vi "fit1.vi"(0 "array":dbl[][](array[numeric]), 5 "num X samples":i32=100, 7 "num Y samples":i32=50, 9 "parameter bounds":T1={"parameter minimum"=[1.0, 0.0, 1.0, 0.0, 1.0, 0.0], "parameter maximum"=[255.0, 640.0, 40.0, 480.0, 40.0, 128.0]}) -> (2 "number of function calls":i32, 3 "Time":u32, 4 "best nonlinear fit":dbl[](array[numeric]), 6 "best fit parameters":dbl[](array[numeric]), 10 "residue":dbl, 14 "estimated parameters":dbl[](array[numeric]), 15 "error out":errorcluster)   [LabVIEW 2015]
uses:
  <vilib>/Analysis/6fits.llb/Curve Fitting Criteria.ctl
  <vilib>/Analysis/1siggen.llb/Ramp Pattern by Samples.vi
  <vilib>/gmath/NumericalOptimization/Nonlinear Curve Fit LM bound.vi
  <vilib>/Analysis/NI_AALBase.lvlib
  <vilib>/gmath/NI_Gmath.lvlib
  <vilib>/Analysis/NI_AALPro.lvlib
panel:
  in  "initial Sigma":dbl=5.0
  out "1D data and fit":dbl[][](graph)
  out "fit param size":i32
  out "Y size":i32
  out "size(bild)":i32[](array[numeric])
  in  "error in (no error)":errorcluster
  in  "termination":cluster{"max iteration":i32, "tolerance":dbl}={"max iteration"=200, "tolerance"=1e-08}
  # "Amplitude"
  # "m1 (Mean 1)"
  # "Sigma 1"
  # "m2 (Mean 2)"
  # "Sigma 2"
  # "Offset"
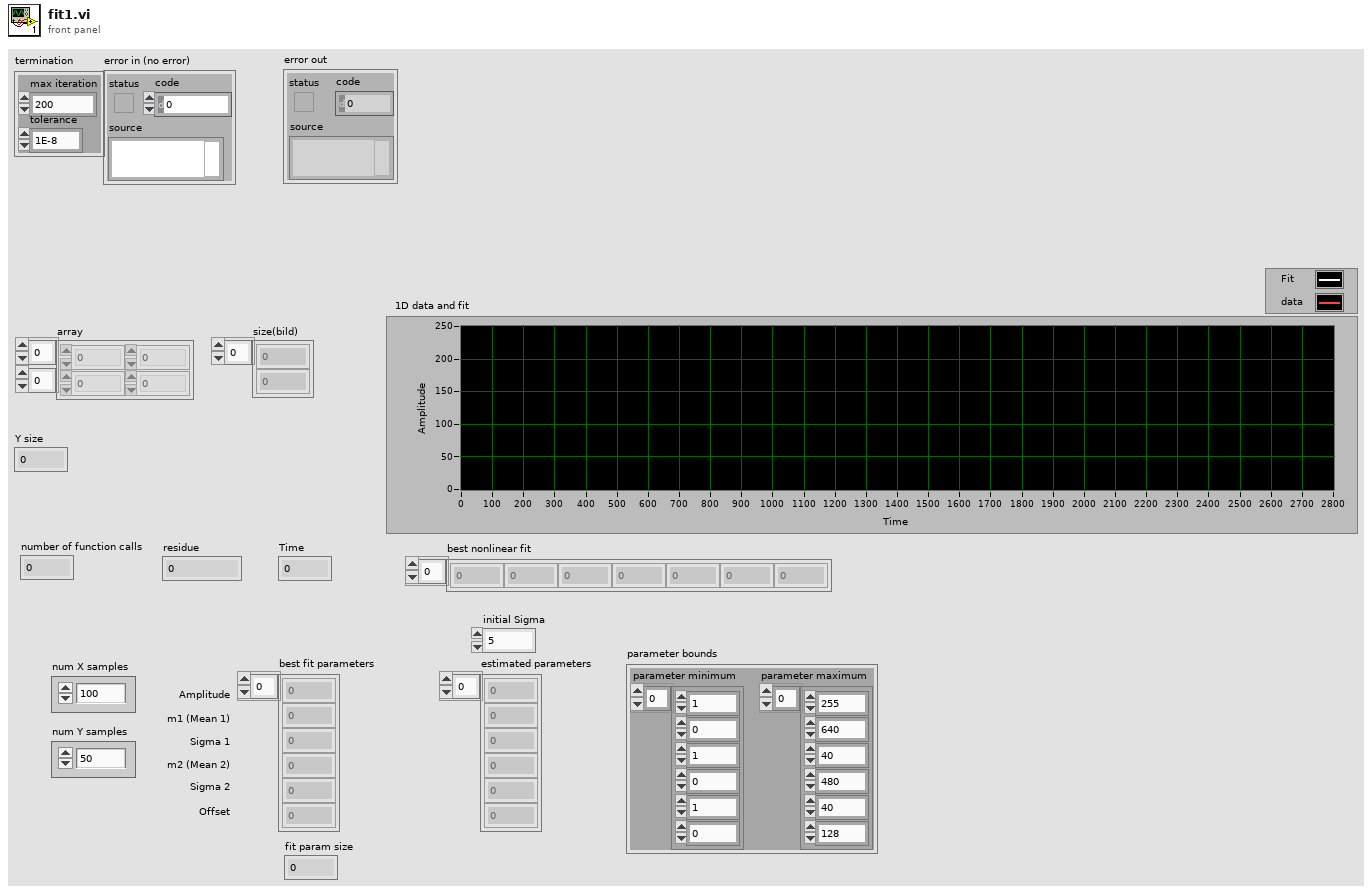
[diagram p1: front panel]
types:
  T1 = cluster{"parameter minimum":dbl[], "parameter maximum":dbl[]}
  T2 = typedef "NI_AALPro.lvlib/Curve Fitting Criteria.ctl" = u16
  T3 = cluster{"num X samples":i32, "num Y samples":i32}
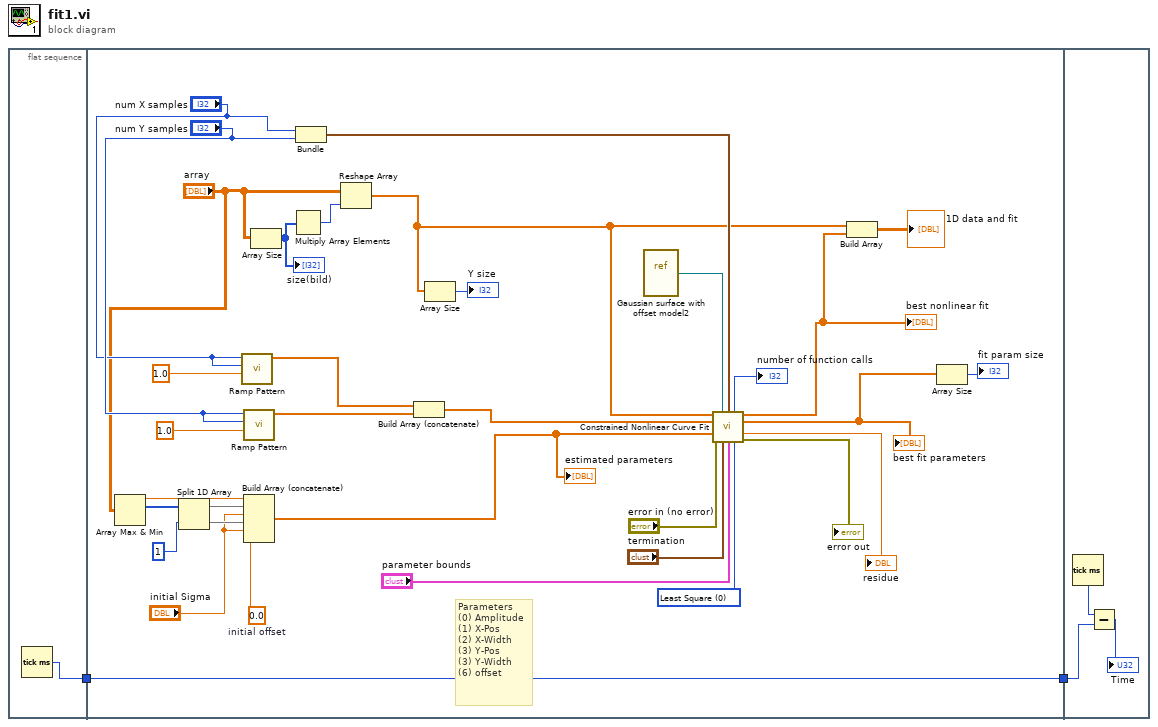
[diagram p0: block diagram]
diagram:
  n1 = flat-sequence {
    tunnel: [w3] -> w2
    tunnel: w2 -> [w37]
    tunnel: [w37] -> w1
    tunnel: w1 -> [w39]
    frame #0 {
      n2 = Tick Count (ms)() -> (millisecond timer value=w3:u32)
    }
    frame #1 {
      w6 = 0.0  # initial offset
      w19 = T2 0 items=["Least Square", "Least Absolute Residual", "Bisquare"] ("method")
      # "Parameters\n(0) Amplitude\n(1) X-Pos\n(2) X-Width\n(3) Y-Pos\n(3) Y-Width\n(6) offset"
      n3 = Array Max & Min(array="array") -> (max value=w13:dbl, max index (indices)=w10:i32[])  [unwired: 2 out]
      n4 = Split 1D Array(array=w10, index=1) -> (first subarray=w9:i32[], second subarray=w8:i32[])
      n5 = call-poly <vilib>:"Ramp Pattern.vi"("start"=1.0, "end"="num X samples", "samples"="num X samples") -> ("Ramp Pattern"=w36:dbl[])  [unwired: 7 in, 1 out]
      n6 = call-poly <vilib>:"Ramp Pattern.vi"("start"=1.0, "end"="num Y samples", "samples"="num Y samples") -> ("Ramp Pattern"=w35:dbl[])  [unwired: 7 in, 1 out]
      n7 = Build Array (concatenate)(w13, w9, "initial Sigma", w8, "initial Sigma", w6) -> (w5:dbl[])
      "estimated parameters" <- w5
      n8 = Array Size(array="array") -> (size(s)=w18:i32[])
      "size(bild)" <- w18
      n9 = Multiply Array Elements(1:w18) -> (0:w17:i32)
      n10 = Bundle("num X samples"="num X samples", "num Y samples"="num Y samples") -> (w24:T3)  [unwired: 1 out]
      n11 = Reshape Array("array", w17) -> (w15:dbl[])
      n12 = Build Array (concatenate)(w36, w35) -> (w20:dbl[])
      n13 = Array Size(array=w15) -> (size(s)=→"Y size":i32)
      n14 = vi-ref "Gaussian surface with offset model2.vi"() -> (w21:refnum<vi>)
      n15 = call-poly <vilib>:"Constrained Nonlinear Curve Fit.vi"("Y"=w15, "f(x,a)"=w21, "data"=w24, "X"=w20, "initial parameters"=w5, "error in (no error)"="error in (no error)", "termination"="termination", "parameter bounds"="parameter bounds", "method"=w19) -> ("number of function calls"=→"number of function calls":i32, "best nonlinear fit"=w14:dbl[], "best fit parameters"=w29:dbl[], "residue"=→"residue":dbl, "error out"=→"error out":errorcluster)  [unwired: 1 in, 1 out]
      "best fit parameters" <- w29
      "best nonlinear fit" <- w14
      n16 = Build Array(w15, w14) -> (→"1D data and fit":dbl[][])
      n17 = Array Size(array=w29) -> (size(s)=→"fit param size":i32)
    }
    frame #2 {
      n18 = Tick Count (ms)() -> (millisecond timer value=w40:u32)
      n19 = Subtract(x=w40, y=w39) -> (x-y=→"Time":u32)
    }
  }
